vi "All RUNs Completed.vi"(8 "error in (no error)":errorcluster, 11 "Monkey in":refnum<class "Monkey.lvclass">) -> (0 "error out":errorcluster, 2 "Monkey Status":T1=enum."Ongoing", 3 "Monkey out":refnum<class "Monkey.lvclass">)   [LabVIEW 2020, in "CIRCUS_uServices.lvlib" / "Monkey.lvlib" / "Monkey.lvclass"]
doc: "Clear Current RUN. Pop-up message saying the RUNs are completed. Change global RUN led status"
uses:
  Monkey.lvclass
  Monkey.lvclass/Monkey.ctl
  Monkey Consumer Case Selector.ctl
  Run Utilities/TypeDefs/Monkey Status.ctl
  Run Utilities/Run Utilities.lvlib
  TALOS/TALOS_PPL.lvlibp/Father of all uServices/Father of all uServices/Father of all uServices.lvclass
  C:/Users/marco/Documents/GitHub_Lab/CIRCUS/TALOS/TALOS_PPL.lvlibp/Father of all uServices/Father of all uServices/Father of all uServices.lvclass
  C:/Users/marco/Documents/GitHub_Lab/CIRCUS/TALOS/TALOS_PPL.lvlibp/Ancestor/Ancestor/Ancestor.lvclass
  C:/Users/marco/Documents/GitHub_Lab/CIRCUS/TALOS/Actor Framework.lvlibp/1abvi3w/vi.lib/ActorFramework/Actor/Actor.lvclass
  C:/Users/marco/Documents/GitHub_Lab/CIRCUS/CIRCUS uServices et al/Monkey/Monkey.lvclass
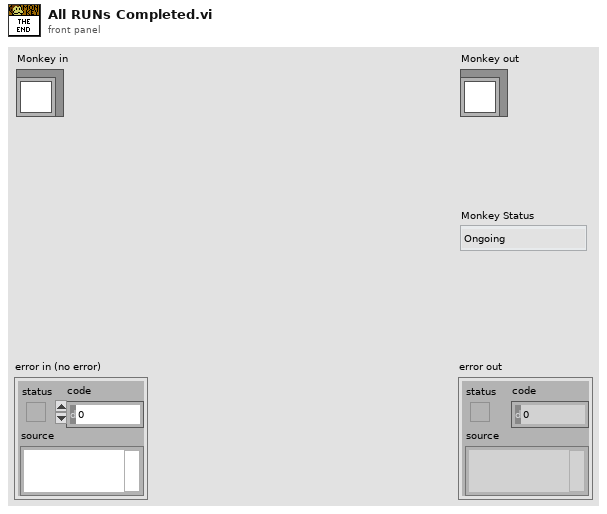
[diagram p1: front panel]
types:
  T1 = typedef "CIRCUS_uServices.lvlib/Run Utilities.lvlib/Monkey Status.ctl" = enum16{"Init", "Paused", "Ongoing", "Stopped", "Finished (no errors)", "Finished (with errors)"}
  T2 = typedef "CIRCUS_uServices.lvlib/Monkey.lvlib/Monkey.lvclass/Monkey Consumer Case Selector.ctl" = enum16{"Init", "Update GUI", "New schedule", "Check Script", "Submit Script", "Banana arrived", "Optimiser - evaluate RUN", "Optimiser - update RUN", "Quality Check", "What to do next", "Update Crit Lvl", "Skip Run", "Stop Schedule", "Skip schedule"}
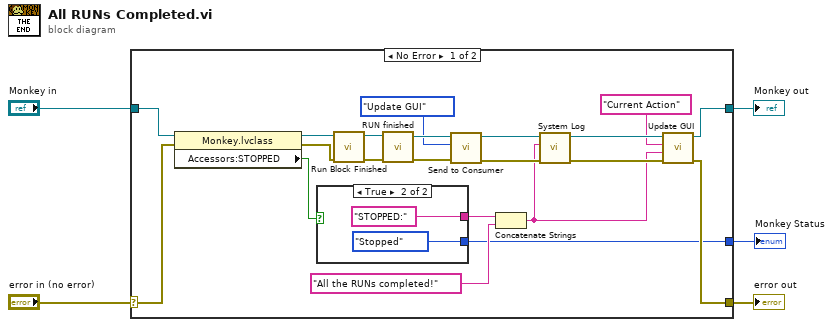
[diagram p0: block diagram]
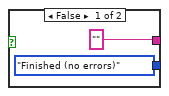
[diagram p2: hidden frame]
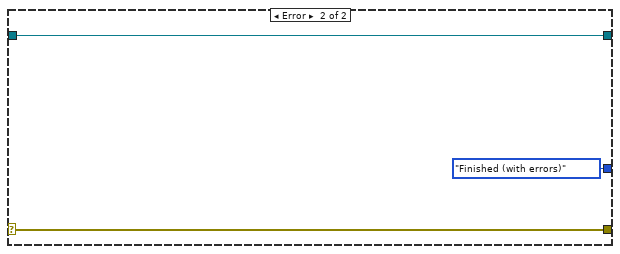
[diagram p3: hidden frame]
diagram:
  n1 = case shown="No Error" "error in (no error)" {
    selector: "error in (no error)" -> [w11 w33]
    tunnel: [w18 w33] -> w4
    tunnel: [w19 w32] -> w2
    tunnel: "Monkey in" -> [w12 w32]
    tunnel: [w16 Monkey_Status."Finished (with errors)" ("Monkey Status")] -> w1
    frame No Error {
      n2 = property class="Monkey.lvclass"(reference=w12, error in=w11) -> (reference out=w10:refnum<class "Monkey.lvclass">, error out=w9:errorcluster, "Accessors:STOPPED"=w14:bool)
      n3 = case shown="True" w14 {
        tunnel: ["" "STOPPED:" ("t")] -> w17
        tunnel: [Monkey_Status."Finished (no errors)" ("Monkey Status") Monkey_Status."Stopped" ("Monkey Status")] -> w16
        frame False {
        }
        frame True {
        }
      }
      n4 = call-dynamic "Run Block Finished.vi"("error in (no error)"=w9, "Monkey in"=w10) -> ("error out"=w7:errorcluster, "Monkey out"=w8:refnum<class "Monkey.lvclass">)  [unwired: 8 in]
      n5 = call-dynamic "RUN finished.vi"("error in (no error)"=w7, "Monkey in"=w8) -> ("error out"=w20:errorcluster, "Monkey out"=w13:refnum<class "Monkey.lvclass">)  [unwired: 8 in]
      n6 = call "Send to Consumer.vi"("error in (no error)"=w20, "Case ID"=Monkey_Consumer_Case_Selector."Update GUI" ("Consumer Case Selector"), "uService Template in"=w13) -> ("error out"=w22:errorcluster, "uService Template out"=w23:refnum<class "Monkey.lvclass">)  [unwired: 7 in]
      n7 = Concatenate Strings(w17, "All the RUNs completed!" ("Text to log")) -> (w15:string)
      n8 = call "System Log.vi"("error in (no error)"=w22, "Text to log"=w15, "uService Template in"=w23) -> ("error out"=w24:errorcluster, "uService Template out"=w26:refnum<class "Monkey.lvclass">)  [unwired: 7 in]
      n9 = call "Update GUI.vi"("error in (no error)"=w24, "Data"=w15, "GUI Item Name"="Current Action", "uService Template in"=w26) -> ("error out"=w18:errorcluster, "uService Template out"=w19:refnum<class "Monkey.lvclass">)  [unwired: 6 in]
    }
    frame Error {
    }
  }
  "error out" <- w4
  "Monkey out" <- w2
  "Monkey Status" <- w1
